vi "Teleop.vi"() -> ()   [LabVIEW 2014]
doc: "This VI is called for each TeleOp packet received from the DS where the robot is not disabled. It is often used to read from the joysticks and update I/O or to update setpoints for timed control loops. It should complete and return within 20 milliseconds or it may miss DS packets."
uses:
  Robot Global Data.vi
panel:
  out "Drive Controller":T1
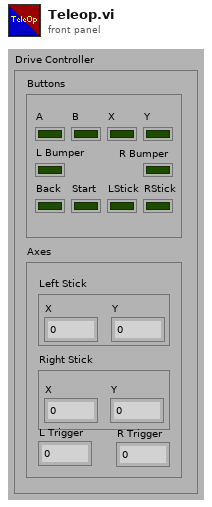
[diagram p1: front panel]
types:
  T1 = cluster{"Buttons":cluster{"A":bool, "B":bool, "X":bool, "Y":bool, "L Bumper":bool, "R Bumper":bool, "Back":bool, "Start":bool, "LStick":bool, "RStick":bool}, "Axes":cluster{"Left Stick":cluster{"X":dbl, "Y":dbl}, "Right Stick":cluster{"X":dbl, "Y":dbl}, "L Trigger":dbl, "R Trigger":dbl}}
  T2 = cluster{"Pickup Mechanism":cluster{"Lift":cluster{"Top":bool, "3":bool, "2":bool, "1":bool, "Bottom":bool}, "Clamp":cluster{"Widest":bool, "Narrowest":bool, "Left Arm":bool, "Right Arm":bool}}, "Ultrasonic":dbl, "Clamper Wide Tote":bool, "Tote in?":bool, "Lift Encoder":cluster{"Distance":dbl, "Rate":dbl, "Direction":bool, "Stopped":bool}, "Drive Encoders":cluster{"Distance":dbl, "Rate":dbl, "Direction":bool, "Stopped":bool}[], "Encoder Distance":dbl}
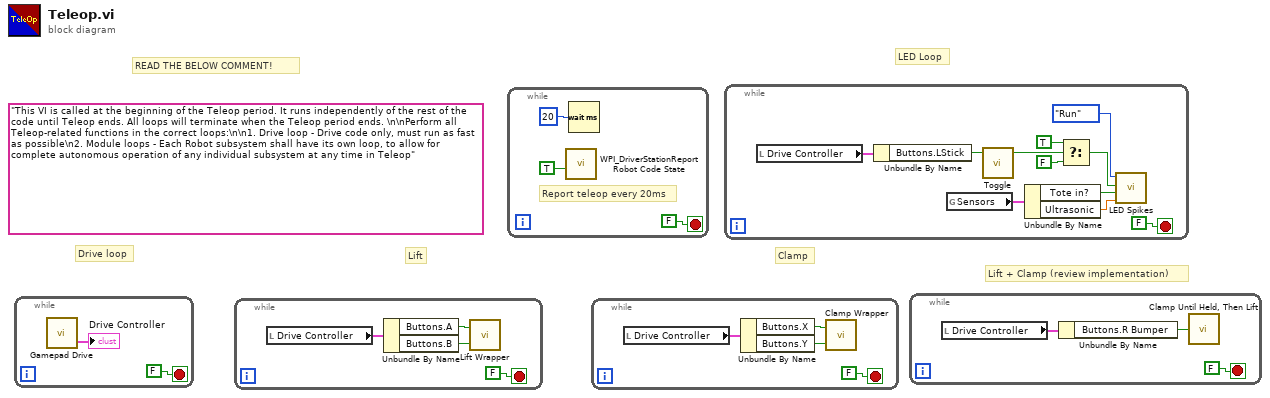
[diagram p0: block diagram]
diagram:
  (unwired) "This VI is called at the beginning of the Teleop period. It runs independently of the rest of the code until Teleop ends. All loops will terminate when the Teleop period ends. \n\nPerform all Teleop-related functions in the correct loops:\n\n1. Drive loop - Drive code only, must run as fast as possible\n2. Module loops - Each Robot subsystem shall have its own loop, to allow for complete autonomous operation of any individual subsystem at any time in Teleop"
  # "Lift + Clamp (review implementation)"
  # "READ THE BELOW COMMENT!"
  # "Clamp"
  # "Lift"
  # "LED Loop"
  # "Drive loop"
  n1 = while {
    stop <- FALSE stop-if-true
    n2 = call "Gamepad Drive.vi"() -> ("XBox"=→"Drive Controller":T1)  [unwired: 3 in]
  }
  n3 = while {
    stop <- FALSE stop-if-true
    n4 = local read "Drive Controller"() -> (w5:T1)
    n5 = Unbundle By Name(w5) -> ("Buttons.A"=w4:bool, "Buttons.B"=w3:bool)
    n6 = call "Lift Wrapper.vi"("Down"=w3, "Up"=w4) -> ()  [unwired: 1 in]
  }
  n7 = while {
    stop <- FALSE stop-if-true
    # "Report teleop every 20ms"
    n8 = call <vilib>:"WPI_DriverStationReport Robot Code State.vi"("TeleOp"=TRUE ("Autonomous")) -> ()  [unwired: 10 in, 1 out]
    n9 = Wait (ms)(milliseconds to wait=u32 20) -> ()  [unwired: 1 out]
  }
  n10 = while {
    stop <- FALSE stop-if-true
    n11 = local read "Drive Controller"() -> (w12:T1)
    n12 = Unbundle By Name(w12) -> ("Buttons.X"=w10:bool, "Buttons.Y"=w11:bool)
    n13 = call "Clamp Wrapper.vi"("In"=w11, "Out"=w10) -> ()  [unwired: 1 in]
  }
  n14 = while {
    stop <- FALSE stop-if-true
    n15 = local read "Drive Controller"() -> (w17:T1)
    n16 = Unbundle By Name(w17) -> ("Buttons.LStick"=w18:bool)
    n17 = global read "Robot Global Data.vi" "Sensors"() -> (w16:T2)
    n18 = call "Toggle.vi"("Input"=w18) -> ("Output"=w19:bool)  [unwired: 4 in]
    n19 = Unbundle By Name(w16) -> ("Tote in?"=w15:bool, "Ultrasonic"=w14:dbl)
    n20 = Select(t=TRUE ("A"), s=w19, f=FALSE ("A")) -> (s? t:f=w20:bool)
    n21 = call "LED Spikes.vi"("Ultrasonic Distance"=w14, "Tote Beam Breaker"=w15, "Camera LED ON/OFF"=w20, "Mode"=enum8{"Start", "Run", "Finish"}."Run") -> ()
  }
  n22 = while {
    stop <- FALSE stop-if-true
    n23 = local read "Drive Controller"() -> (w26:T1)
    n24 = Unbundle By Name(w26) -> ("Buttons.R Bumper"=w25:bool)
    n25 = call "Clamp Until Held, Then Lift.vi"("Clamp + Lift"=w25) -> ()
  }
